vi "example Ver2.vi"() -> ()   [LabVIEW 2023]
uses:
  gfitsio.lvlib
  <vilib>/picture/picture.llb/Draw True-Color Pixmap.vi
  gfitsio-read-image-subset-i32-2d.vi
  gfitsio-write-image-subset-i32-2d.vi
  cfitsio-bitpix.ctl
panel:
  in  "path 2":path=path "C:/OCI-FPA-LabVIEW/Drivers/GFITSIO/sandbox/nasa.bmp"
  out "size(s)":i32[](array[numeric])=[450, 570]
  out "path":path=path "C:/OCI-FPA-LabVIEW/Drivers/GFITSIO/sandbox/nasa.bmp.fits"
  out "Green":picture
  out "Red":picture
  out "Blue":picture
  out "hdu name (dialog if empty)":string
  out "hdu names":string[](array[string])=["Primary", "nasa.bmp"]
  out "hdu name":string="nasa.bmp"
  in  "Tab Control":enum32{"Complete Image", "Red", "Green", "Blue"}(tab)
  out "Complete Image":picture
  # "Run the VI to create a FITS file from a BMP image stored on disk and then read back the FITS file to populate the image below."
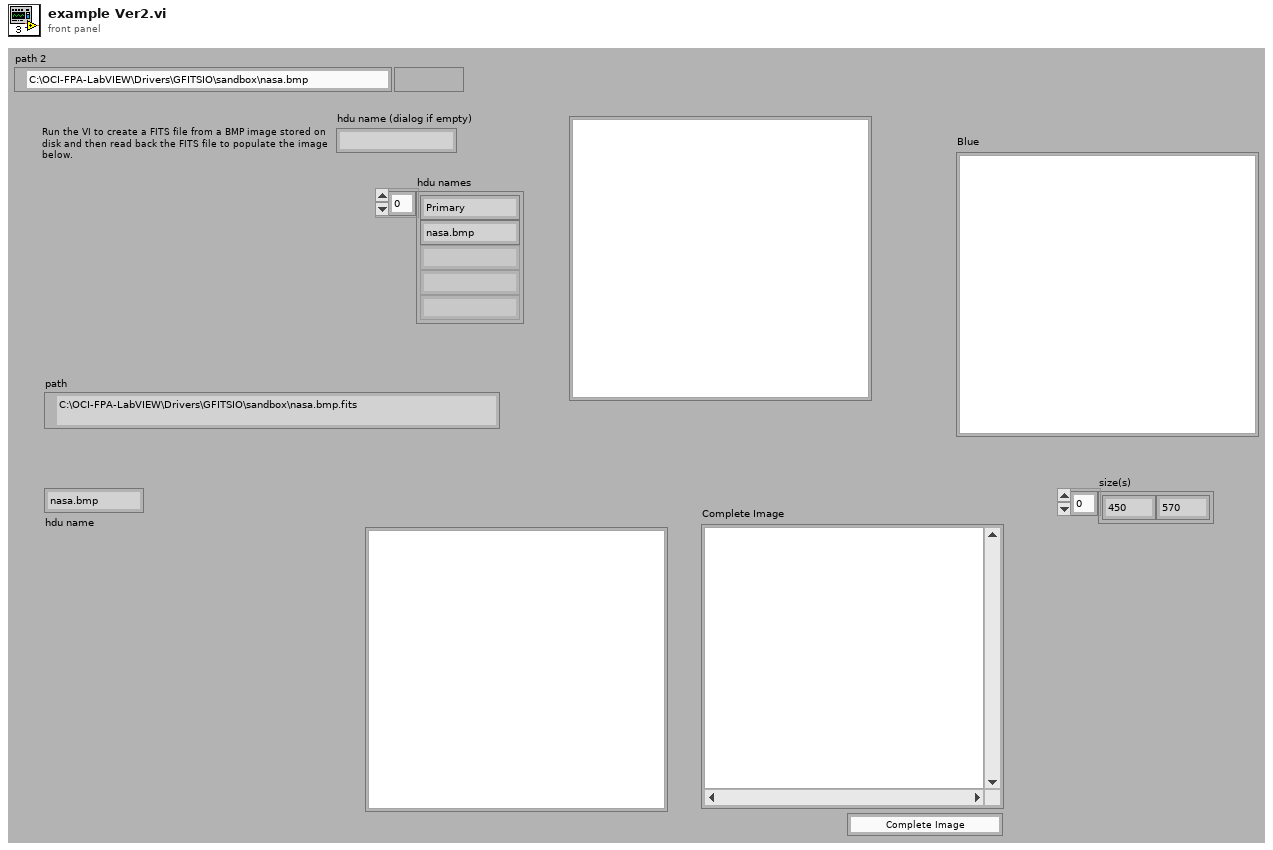
[diagram p1: front panel]
types:
  T1 = enum16{"open", "open or create", "create", "create or replace"}
  T2 = enum16{"open", "open or create", "create or replace", "create", "open (read only)"}
  T3 = typedef "gfitsio.lvlib/cfitsio-bitpix.ctl" = i32
  T4 = typedef "imagedata.ctl" = cluster{"image type":i32, "image depth":i32, "image":u8[], "mask":u8[], "colors":u32[], "Rectangle":cluster{"left":i16, "top":i16, "right":i16, "bottom":i16}}
  T5 = typedef "gfitsio.lvlib/gfitsio-refnum.ctl" = refnum<k1>
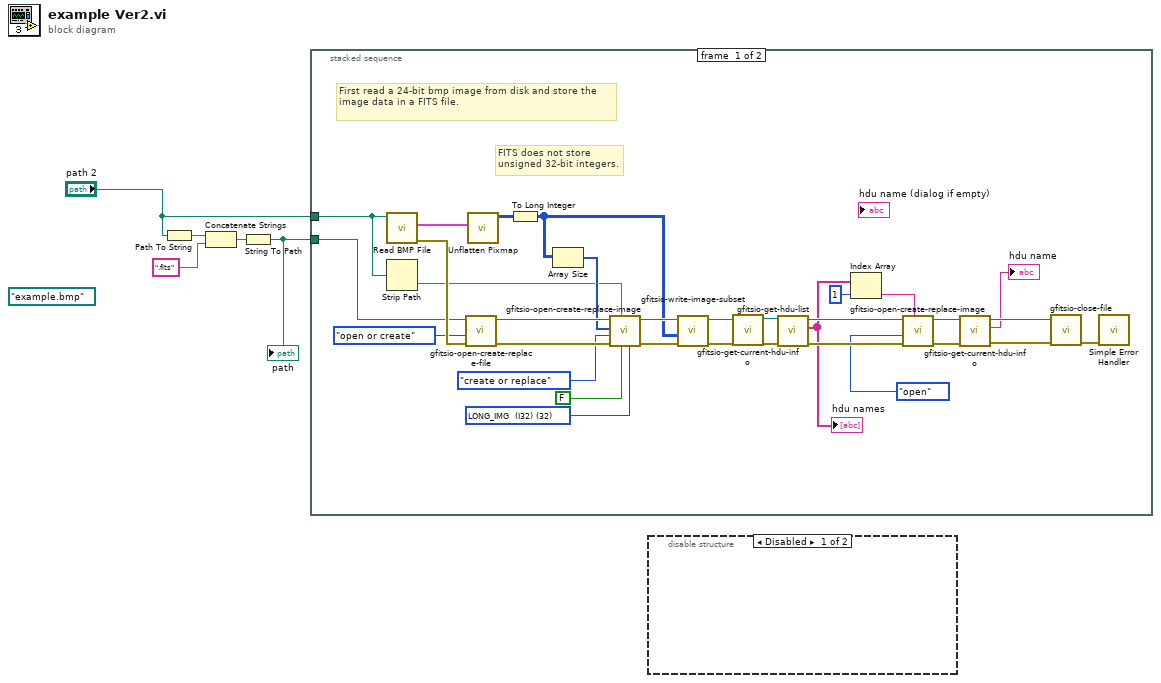
[diagram p0: block diagram]
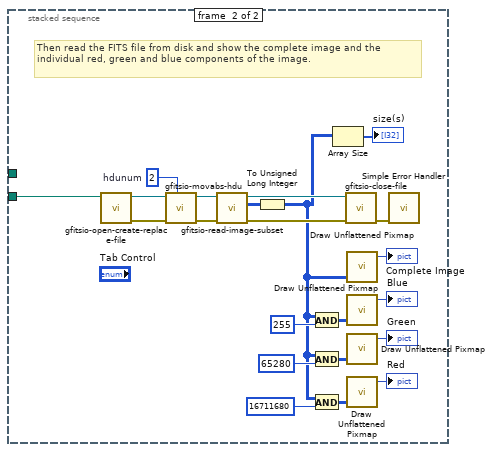
[diagram p3: hidden frame]
diagram:
  (unwired) path "example.bmp" ("path to BMP file")
  n1 = Path To String(path="path 2") -> (string=w3:string)
  n2 = Concatenate Strings(w3, ".fits" ("string")) -> (w5:string)
  n3 = String To Path(string=w5) -> (path=w2:path)
  "path" <- w2
  n4 = stacked-sequence {
    tunnel: "path 2" -> [w22 _]
    tunnel: w2 -> [w23 w40]
    frame #0 {
      w27 = T3 32 items=["<invalid type>"=0, "BYTE_IMG  (U8)"=8, "SHORT_IMG  (I16)"=16, "USHORT_IMG  (U16)"=20, "LONG_IMG  (I32)"=32, "ULONG_IMG  (U32)"=40, "FLOAT_IMG  (SGL)"=-32, "DOUBLE_IMG  (DBL)"=-64] ("image data type")
      # "First read a 24-bit bmp image from disk and store the image data in a FITS file."
      # "FITS does not store unsigned 32-bit integers."
      n5 = call <vilib>:"Read BMP File.vi"("path to BMP file"=w22) -> ("error out"=w33:errorcluster, "image data"=w26:T4)  [unwired: 8 in, 1 out]
      n6 = Strip Path(path=w22) -> (name=w21:string)  [unwired: 1 out]
      n7 = call "gfitsio-open-create-replace-file.vi"("error in (no error)"=w33, "function (open)"=T2."open or create", "file path (dialog if empty)"=w23) -> ("error out"=w36:errorcluster, "gfits refnum"=w37:T5)  [unwired: 6 in, 1 out]
      n8 = call <vilib>:"Unflatten Pixmap.vi"("image data"=w26) -> ("24-bit pixmap"=w32:u32[][])  [unwired: 4 in, 6 out]
      n9 = To Long Integer(number=w32) -> (32bit integer=w29:i32[][])
      n10 = Array Size(array=w29) -> (size(s)=w28:i32[])
      n11 = call "gfitsio-open-create-replace-image.vi"("image data type"=w27, "advisory dialog? (display:T)"=FALSE, "hdu name (dialog if empty)"=w21, "error in (no error)"=w36, "function (create or replace)"=T1."create or replace" ("function (open or create)"), "naxes"=w28, "gfits refnum"=w37) -> ("error out"=w35:errorcluster, "dup gfits refnum"=w34:T5)  [unwired: 2 in, 1 out]
      n12 = call-poly "gfitsio-write-image-subset.vi"("error in (no error)"=w35, "data"=w29, "gfits refnum"=w34) -> ("error out"=w19:errorcluster, "dup gfits refnum"=w20:T5)  [unwired: 7 in]
      n13 = call "gfitsio-get-current-hdu-info.vi"("error in (no error)"=w19, "gfits refnum"=w20) -> ("error out"=w17:errorcluster, "dup gfits refnum"=w18:T5)  [unwired: 5 in, 3 out]
      n14 = call "gfitsio-get-hdu-list.vi"("error in (no error)"=w17, "gfits refnum"=w18) -> ("error out"=w15:errorcluster, "hdu names"=w8:string[], "dup gfits refnum"=w16:T5)  [unwired: 6 in, 1 out]
      "hdu names" <- w8
      n15 = Index Array(array=w8, index=1) -> (element=w7:string)
      n16 = call "gfitsio-open-create-replace-image.vi"("hdu name (dialog if empty)"=w7, "error in (no error)"=w15, "function (create or replace)"=T1."open", "gfits refnum"=w16) -> ("error out"=w12:errorcluster, "dup gfits refnum"=w13:T5)  [unwired: 5 in, 1 out]
      n17 = call "gfitsio-get-current-hdu-info.vi"("error in (no error)"=w12, "gfits refnum"=w13) -> ("error out"=w10:errorcluster, "hdu name"=→"hdu name":string, "dup gfits refnum"=w11:T5)  [unwired: 5 in, 2 out]
      n18 = call "gfitsio-close-file.vi"("error in (no error)"=w10, "gfits refnum"=w11) -> ("error out"=w25:errorcluster)  [unwired: 8 in, 1 out]
      n19 = call <vilib>:"Simple Error Handler.vi"("error in (no error)"=w25) -> ()  [unwired: 4 in, 5 out]
    }
    frame #1 {
      w52 = 2  # hdunum
      # "Then read the FITS file from disk and show the complete image and the individual red, green and blue components of the image."
      n20 = call "gfitsio-open-create-replace-file.vi"("file path (dialog if empty)"=w40) -> ("error out"=w59:errorcluster, "gfits refnum"=w58:T5)  [unwired: 8 in, 1 out]
      n21 = call "gfitsio-movabs-hdu.vi"("hdunum"=w52, "error in (no error)"=w59, "gfits refnum"=w58) -> ("error out"=w57:errorcluster, "dup gfits refnum"=w56:T5)  [unwired: 6 in, 1 out]
      n22 = call-poly "gfitsio-read-image-subset.vi"("error in (no error)"=w57, "gfits refnum"=w56) -> ("error out"=w55:errorcluster, "data"=w51:i32[][], "dup gfits refnum"=w54:T5)  [unwired: 7 in]
      n23 = To Unsigned Long Integer(number=w51) -> (unsigned 32bit integer=w39:u32[][])
      n24 = And(x=w39, y=u32 255) -> (x .and. y?=w47:u32[][])
      n25 = And(x=w39, y=u32 65280) -> (x .and. y?=w44:u32[][])
      n26 = And(x=w39, y=u32 16711680) -> (x .and. y?=w42:u32[][])
      n27 = Array Size(array=w39) -> (size(s)=→"size(s)":i32[])
      n28 = call "gfitsio-close-file.vi"("error in (no error)"=w55, "gfits refnum"=w54) -> ("error out"=w53:errorcluster)  [unwired: 8 in, 1 out]
      n29 = call-poly <vilib>:"Draw Unflattened Pixmap.vi"("data (RGB format)"=w39) -> ("new picture"=→"Complete Image":picture)  [unwired: 8 in]
      n30 = call-poly <vilib>:"Draw Unflattened Pixmap.vi"("data (RGB format)"=w47) -> ("new picture"=→"Blue":picture)  [unwired: 8 in]
      n31 = call-poly <vilib>:"Draw Unflattened Pixmap.vi"("data (RGB format)"=w44) -> ("new picture"=→"Green":picture)  [unwired: 8 in]
      n32 = call-poly <vilib>:"Draw Unflattened Pixmap.vi"("data (RGB format)"=w42) -> ("new picture"=→"Red":picture)  [unwired: 8 in]
      n33 = call <vilib>:"Simple Error Handler.vi"("error in (no error)"=w53) -> ()  [unwired: 4 in, 5 out]
    }
  }
  n34 = disable-structure shown="Disabled" {
    frame Disabled {
    }
    frame Enabled {
    }
  }
